vi "Match All Spara Channel.vi"(9 "Spara Type Channel":string, 10 "Search Channel":string, 11 "Channel Name":string) -> (3 "Load This?":bool)   [LabVIEW 2011]
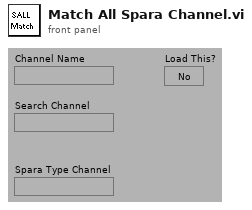
[diagram p1: front panel]
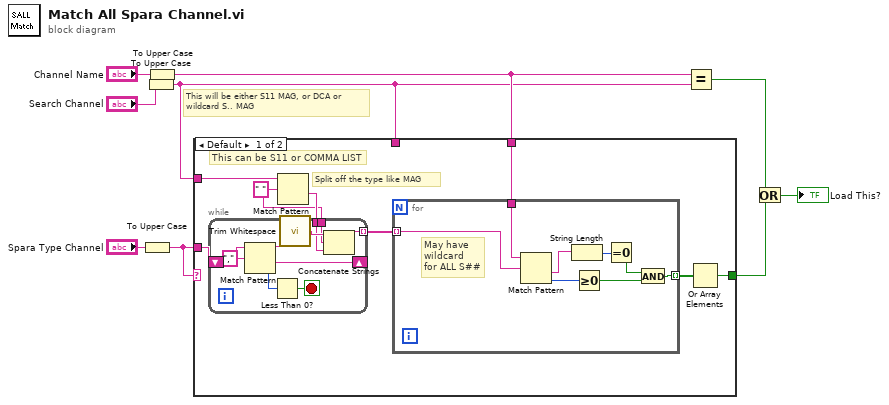
[diagram p0: block diagram]
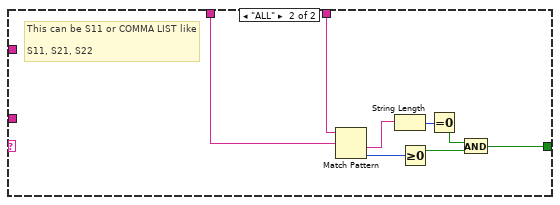
[diagram p2: hidden frame]
diagram:
  # "This will be either S11 MAG, or DCA or\nwildcard S.. MAG"
  n1 = To Upper Case(1:"Spara Type Channel") -> (0:w3:string)
  n2 = To Upper Case(1:"Search Channel") -> (0:w1:string)
  n3 = To Upper Case(1:"Channel Name") -> (0:w7:string)
  n4 = case shown="Default" w3 {
    tunnel: w7 -> [w17 w38]
    tunnel: w3 -> [w13 _]
    tunnel: [w14 w36] -> w5
    tunnel: w1 -> [_ w37]
    tunnel: w1 -> [w12 _]
    frame Default {
      w10 = " " ("regular expression")
      # "Split off the type like MAG"
      # "This can be S11 or COMMA LIST"
      n5 = Match Pattern(string=w12, regular expression=w10) -> (after substring=w11:string)  [unwired: 4 out]
      n6 = while {
        shift-right: [w30] -> _
        shift-left: w13 -> [w35]
        tunnel: [w28] -> w15 mode=indexing
        tunnel: w11 -> [w27]
        tunnel: w10 -> [w26]
        stop <- w32 stop-if-true
        n7 = Match Pattern(string=w35, regular expression=",") -> (before substring=w33:string, after substring=w30:string, offset past match=w31:i32)  [unwired: 2 out]
        n8 = Less Than 0?(x=w31) -> (x < 0?=w32:bool)
        n9 = call <vilib>:"Trim Whitespace.vi"("string"=w33) -> ("trimmed string"=w29:string)  [unwired: 1 in]
        n10 = Concatenate Strings(w29, w26, w27) -> (w28:string)
      }
      n11 = for {
        tunnel: w17 -> [w24]
        tunnel: [w23] -> w16 mode=indexing
        tunnel: w15 -> [w22] mode=indexing
        # "May have \nwildcard\nfor ALL S##"
        n12 = Match Pattern(string=w24, regular expression=w22) -> (after substring=w21:string, offset past match=w25:i32)  [unwired: 3 out]
        n13 = String Length(string=w21) -> (length=w20:i32)
        n14 = Greater Or Equal To 0?(x=w25) -> (x >= 0?=w18:bool)
        n15 = Equal To 0?(x=w20) -> (x = 0?=w19:bool)
        n16 = And(x=w19, y=w18) -> (x .and. y?=w23:bool)
      }
      n17 = Or Array Elements(Boolean array=w16) -> (logical OR=w14:bool)
    }
    frame "ALL" {
      # "This can be S11 or COMMA LIST like\n\nS11, S21, S22"
      n18 = Match Pattern(string=w38, regular expression=w37) -> (after substring=w40:string, offset past match=w39:i32)  [unwired: 3 out]
      n19 = String Length(string=w40) -> (length=w41:i32)
      n20 = Greater Or Equal To 0?(x=w39) -> (x >= 0?=w43:bool)
      n21 = Equal To 0?(x=w41) -> (x = 0?=w42:bool)
      n22 = And(x=w42, y=w43) -> (x .and. y?=w36:bool)
    }
  }
  n23 = Equal?(x=w7, y=w1) -> (x = y?=w9:bool)
  n24 = Or(x=w9, y=w5) -> (x .or. y?=→"Load This?":bool)
